vi "Visa sim.vi"() -> ()   [LabVIEW 2017]
uses:
  <vilib>/Instr/_visa.llb/VISA Open Access Mode.ctl
panel:
  out "Telegram String":string
  out "Distance Array":u32[](array[numeric])
  out "Angle Array":dbl[](array[numeric])
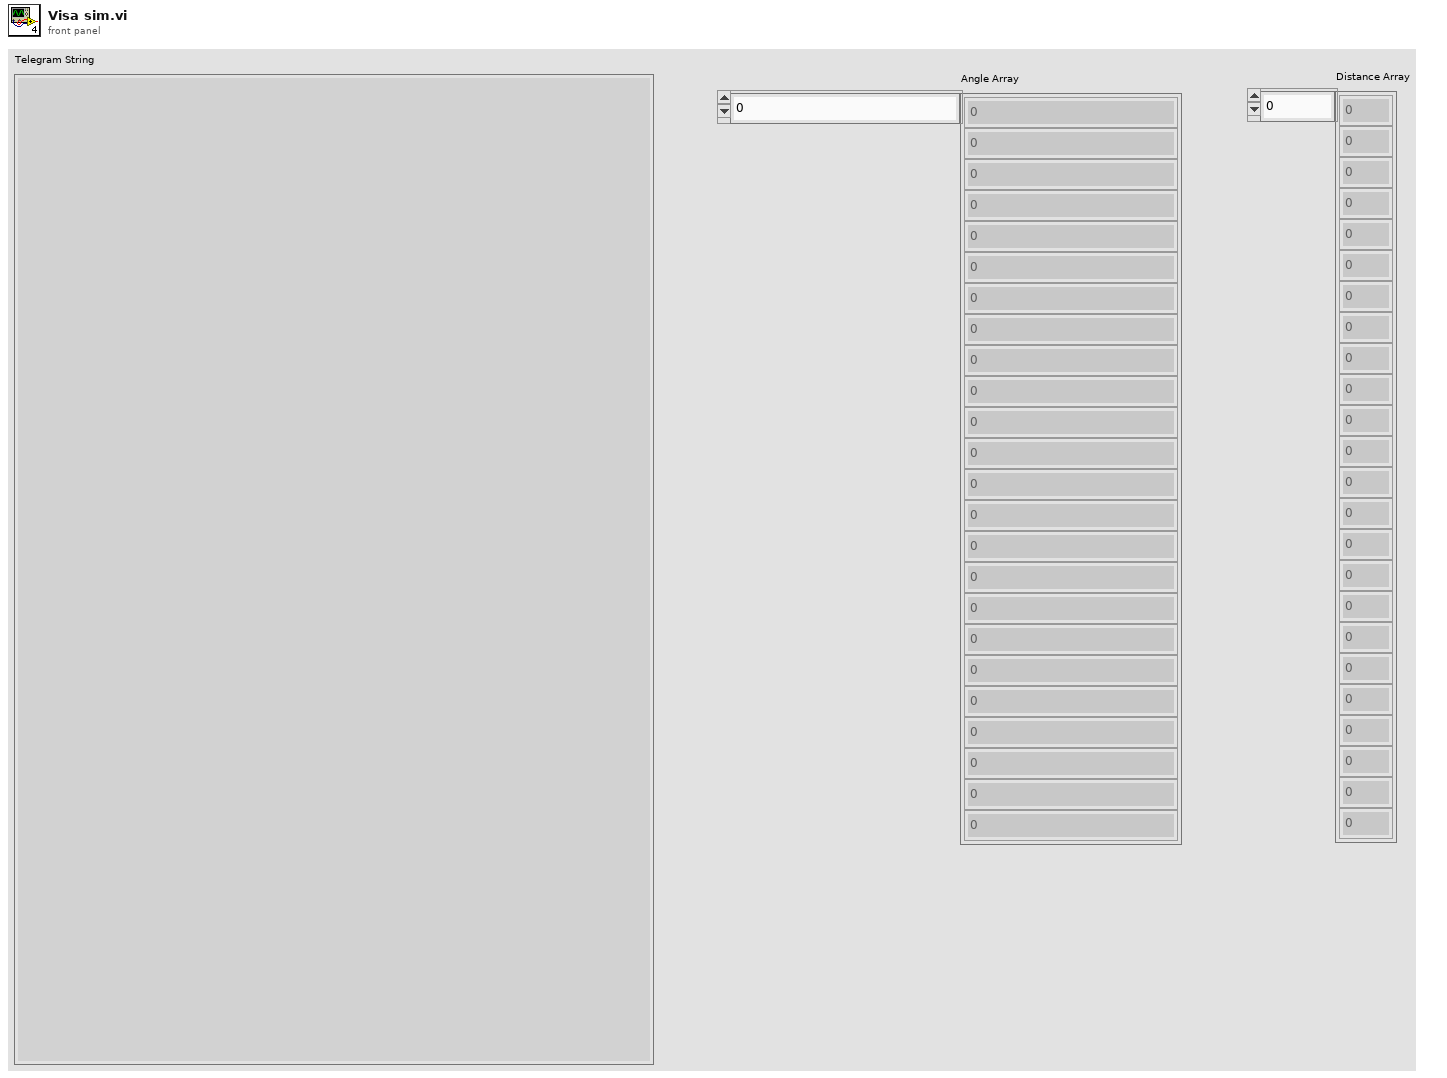
[diagram p1: front panel]
types:
  T1 = typedef "VISA Open Access Mode.ctl" = u32
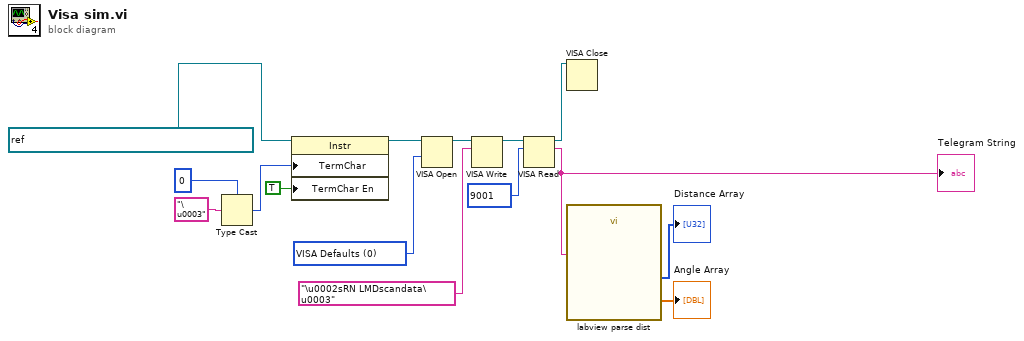
[diagram p0: block diagram]
diagram:
  w8 = T1 0 items=["VISA Defaults"=0, "Exclusive Lock"=1, "Load Configured Settings"=4] ("Access Mode")
  n1 = Type Cast(type=u8 0, x="\u0003") -> (*(type *) &x=w11:u8)
  n2 = property class="Instr"(reference=refnum<visa-resource-name> "TCPIP::169.254.233.170::2112::SOCKET" ("VISA resource name"), "TermChar"=w11, "TermChar En"=TRUE) -> (reference out=w2:refnum<visa-resource-name>)  [unwired: 1 in, 1 out]
  n3 = VISA Open(access mode=w8, VISA resource name=w2) -> (VISA resource name=w7:refnum<visa-resource-name>)  [unwired: 3 in, 1 out]
  n4 = VISA Write(VISA resource name=w7, write buffer="\u0002sRN LMDscandata\u0003") -> (VISA resource name out=w1:refnum<visa-resource-name>)  [unwired: 1 in, 2 out]
  n5 = VISA Read(VISA resource name=w1, byte count=u32 9001) -> (VISA resource name out=w15:refnum<visa-resource-name>, read buffer=w6:string)  [unwired: 1 in, 2 out]
  "Telegram String" <- w6
  n6 = VISA Close(VISA resource name=w15) -> ()  [unwired: 1 in, 1 out]
  n7 = call "labview parse dist.vi"("Telegram String"=w6) -> ("Angle Array"=→"Angle Array":dbl[], "Distance Array"=→"Distance Array":u32[])  [unwired: 8 in]
